vi "close.vi"(8 "error in (no error)":errorcluster, 11 "USB-6000 in":refnum<class "USB-6000.lvclass">) -> (0 "error out":errorcluster, 3 "USB-6000 out":refnum<class "USB-6000.lvclass">)   [LabVIEW 2025, in "USB IO.lvlib" / "USB-6000.lvclass"]
uses:
  USB-6000.lvclass
  USB-6000.lvclass/USB-6000.ctl
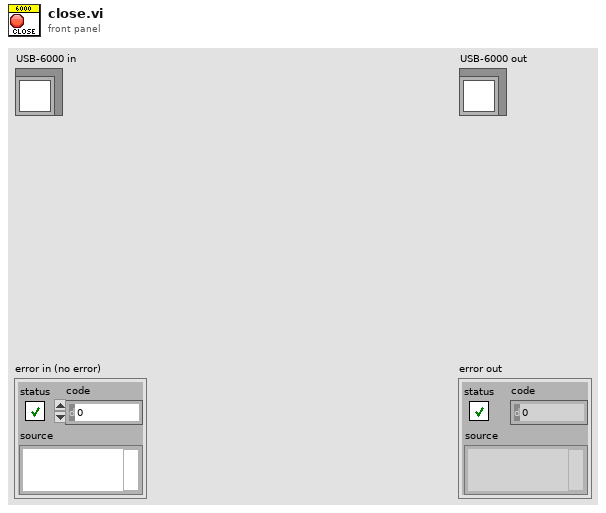
[diagram p1: front panel]
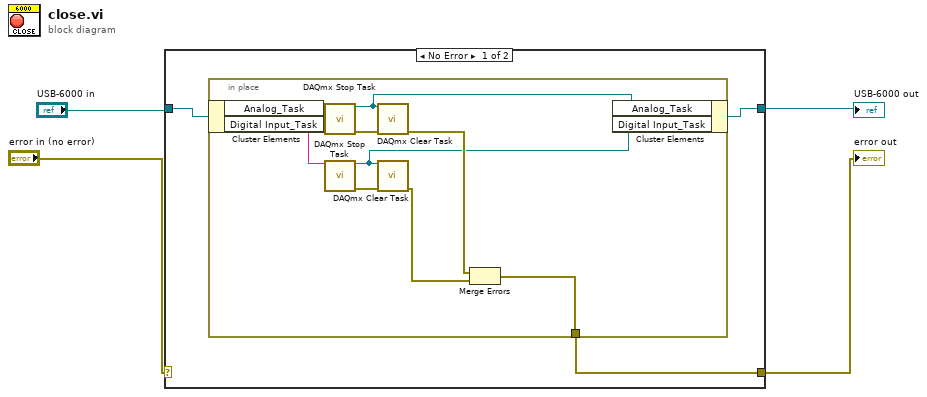
[diagram p0: block diagram]
diagram:
  n1 = case shown="No Error" "error in (no error)" {
    selector: "error in (no error)" -> [_ w18]
    tunnel: [w5 w18] -> w1
    tunnel: [w6 w17] -> w3
    tunnel: "USB-6000 in" -> [w7 w17]
    frame No Error {
      n2 = in-place {
        in-place-border: [w11] -> w5
        n3 = in-place-cluster #1(w7) -> ("Analog_Task"=w16:string, "Digital Input_Task"=w12:string)
        n4 = call <vilib>:"DAQmx Stop Task.vi"("task/channels in"=w16) -> ("task out"=w14:refnum<k21>, "error out"=w15:errorcluster)  [unwired: 13 in]
        n5 = call <vilib>:"DAQmx Stop Task.vi"("task/channels in"=w12) -> ("task out"=w8:refnum<k21>, "error out"=w13:errorcluster)  [unwired: 13 in]
        n6 = call <vilib>:"DAQmx Clear Task.vi"("task in"=w14, "error in"=w15) -> ("error out"=w9:errorcluster)  [unwired: 13 in]
        n7 = call <vilib>:"DAQmx Clear Task.vi"("task in"=w8, "error in"=w13) -> ("error out"=w10:errorcluster)  [unwired: 13 in]
        n8 = Merge Errors(w9, w10) -> (w11:errorcluster)
        n9 = in-place-cluster #1("Analog_Task"=w14, "Digital Input_Task"=w8) -> (w6:refnum<class "USB-6000.lvclass">)
      }
    }
    frame Error {
    }
  }
  "error out" <- w1
  "USB-6000 out" <- w3
